vi "Disconnect.vi"(8 "error in (no error)":errorcluster, 9 "Connection Name":string) -> (0 "error out":errorcluster, 2 "isSshConnected":bool, 3 "Return String":string)   [LabVIEW 2015, in "LabSFTP.lvlib"]
doc: "<License>This software is distributed under the BSD 3-Clause License. For the full license please see license.txt or visit www.labvolution.com/license</License>"
uses:
  LabSFTP.lvlib
  FGV State..enum.ctl
  C:/Working Folder/ssh.git/LabSSH Library/References/LabSFTP.dll
  References/LabSFTP.dll
  <vilib>/Utility/error.llb/Error Cluster From Error Code.vi
  <vilib>/ErrorRing/Error Ring.xnode
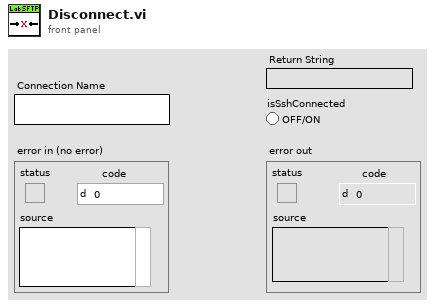
[diagram p1: front panel]
types:
  T1 = typedef "LabSFTP.lvlib/FGV State..enum.ctl" = enum16{"GET", "SET"}
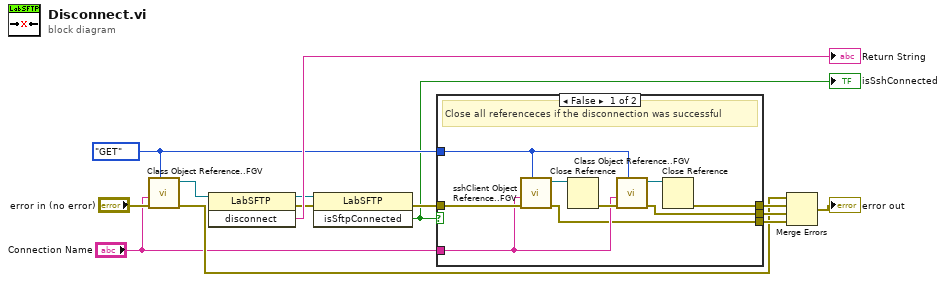
[diagram p0: block diagram]
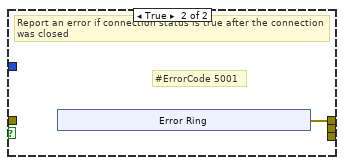
[diagram p2: hidden frame]
diagram:
  w9 = FGV_State..enum."GET" ("FGV State")
  n1 = call "Class Object Reference..FGV.vi"("FGV State"=w9, "error in (no error)"="error in (no error)", "Connection Name"="Connection Name") -> ("error out"=w2:errorcluster, "LabSFTP ref out"=w11:refnum<k24>)  [unwired: 7 in]
  n2 = invoke class="LabSFTP" method="disconnect"(reference=w11) -> (reference out=w7:refnum<k24>, error out=w10:errorcluster, "disconnect"=→"Return String":string)  [unwired: 2 in]
  n3 = invoke class="LabSFTP" method="isSftpConnected"(reference=w7, error in=w10) -> (error out=w8:errorcluster, "isSftpConnected"=w6:bool)  [unwired: 1 in, 1 out]
  "isSshConnected" <- w6
  n4 = case shown="False" w6 {
    tunnel: w9 -> [w23 _]
    tunnel: [w22 w24] -> w13
    tunnel: w8 -> [w19 _]
    tunnel: "Connection Name" -> [w17 _]
    tunnel: [w16 _] -> w4
    tunnel: [w15 _] -> w3
    frame False {
      # "Close all referenceces if the disconnection was successful"
      n5 = call "sshClient Object Reference..FGV.vi"("FGV State"=w23, "error in (no error)"=w19, "Connection Name"=w17) -> ("error out"=w15:errorcluster, "sftpClient ref out"=w20:refnum<k24>)  [unwired: 7 in]
      n6 = Close Reference(reference=w20) -> (error out=w18:errorcluster)  [unwired: 1 in]
      n7 = call "Class Object Reference..FGV.vi"("FGV State"=w23, "error in (no error)"=w18, "Connection Name"=w17) -> ("error out"=w16:errorcluster, "LabSFTP ref out"=w21:refnum<k24>)  [unwired: 7 in]
      n8 = Close Reference(reference=w21) -> (error out=w22:errorcluster)  [unwired: 1 in]
    }
    frame True {
      # "#ErrorCode 5001"
      # "Report an error if connection status is true after the connection was closed"
      n9 = xnode "Error Ring"() -> ("error out"=w24:errorcluster)
    }
  }
  n10 = Merge Errors(w2, w13, w4, w3) -> (→"error out":errorcluster)
